vi "whoilbert -- test -- V1.vi"() -> ()   [LabVIEW 2020]
uses:
  publisher action.ctl
panel:
  in  "sweeper panel 4":enum32{"orig"}(tab)
  out "Plot: wsweep window vs ω  2":cluster{dbl[], dbl[]}[](graph)
  in  "sweeper panel 3":enum32{"wform"}(tab)
  out "Plot: wsweep window vs ω":cluster{dbl[], dbl[]}[](graph)
  in  "scale gauge: Plot: wsweep win 2":dbl(slide)=4644576329.775502 min=0.0 max=0.3 step=1e-06 scale=1e-05..50000000000.0 scale format="%#_3p"
  in  "sweeper panel 2":enum32{"main", "parameters"}(tab)
  out "Plot: wsweep window":cluster{dbl[], dbl[]}[](graph)
  in  "scale gauge: Plot: wsweep win":dbl(slide)=4644576329.775502 min=0.0 max=0.3 step=1e-06 scale=1e-05..1000.0 scale format="%#_3p"
  in  "woffset":dbl(slide)=0.6996996996996996 scale=-10.0..10.0
  in  "wrange":dbl=10000.0 format="%#_13g"
  in  "wpoints":i64=100
  in  "ω1":cdb=0.0-40.0i format="%#_13g"
  in  "ω2":cdb=0.0-1.0i format="%#_13g"
  in  "A1":cdb=2.0+0.0i format="%#_13g"
  in  "A2":cdb=1.0+0.0i format="%#_13g"
  in  "κ0":dbl(slide)=5.830000000000001e-10 min=0.0 max=0.3 step=1e-12 scale=1e-10..1e-07 scale format="%#_3p"
  in  "ζ":dbl(slide)=0.003542 min=0.0 max=0.3 step=1e-06 scale=1e-05..10.0 scale format="%#_3p"
  in  "τN":dbl(slide)=0.004864484047644512 min=0.0 max=0.3 step=1e-06 scale=1e-06..10.0 scale format="%#_3p"
  in  "T1":dbl(slide)=0.03855743450772209 min=0.0 max=0.3 step=1e-06 scale=0.0001..10.0 scale format="%#_3p"
  in  "τC":dbl(slide)=0.09541 min=0.0 max=0.3 step=1e-06 scale=1e-05..10.0 scale format="%#_3p"
  in  "τS":dbl(slide)=0.02006412528739728 min=0.0 max=0.3 step=1e-06 scale=0.001..10.0 scale format="%#_3p"
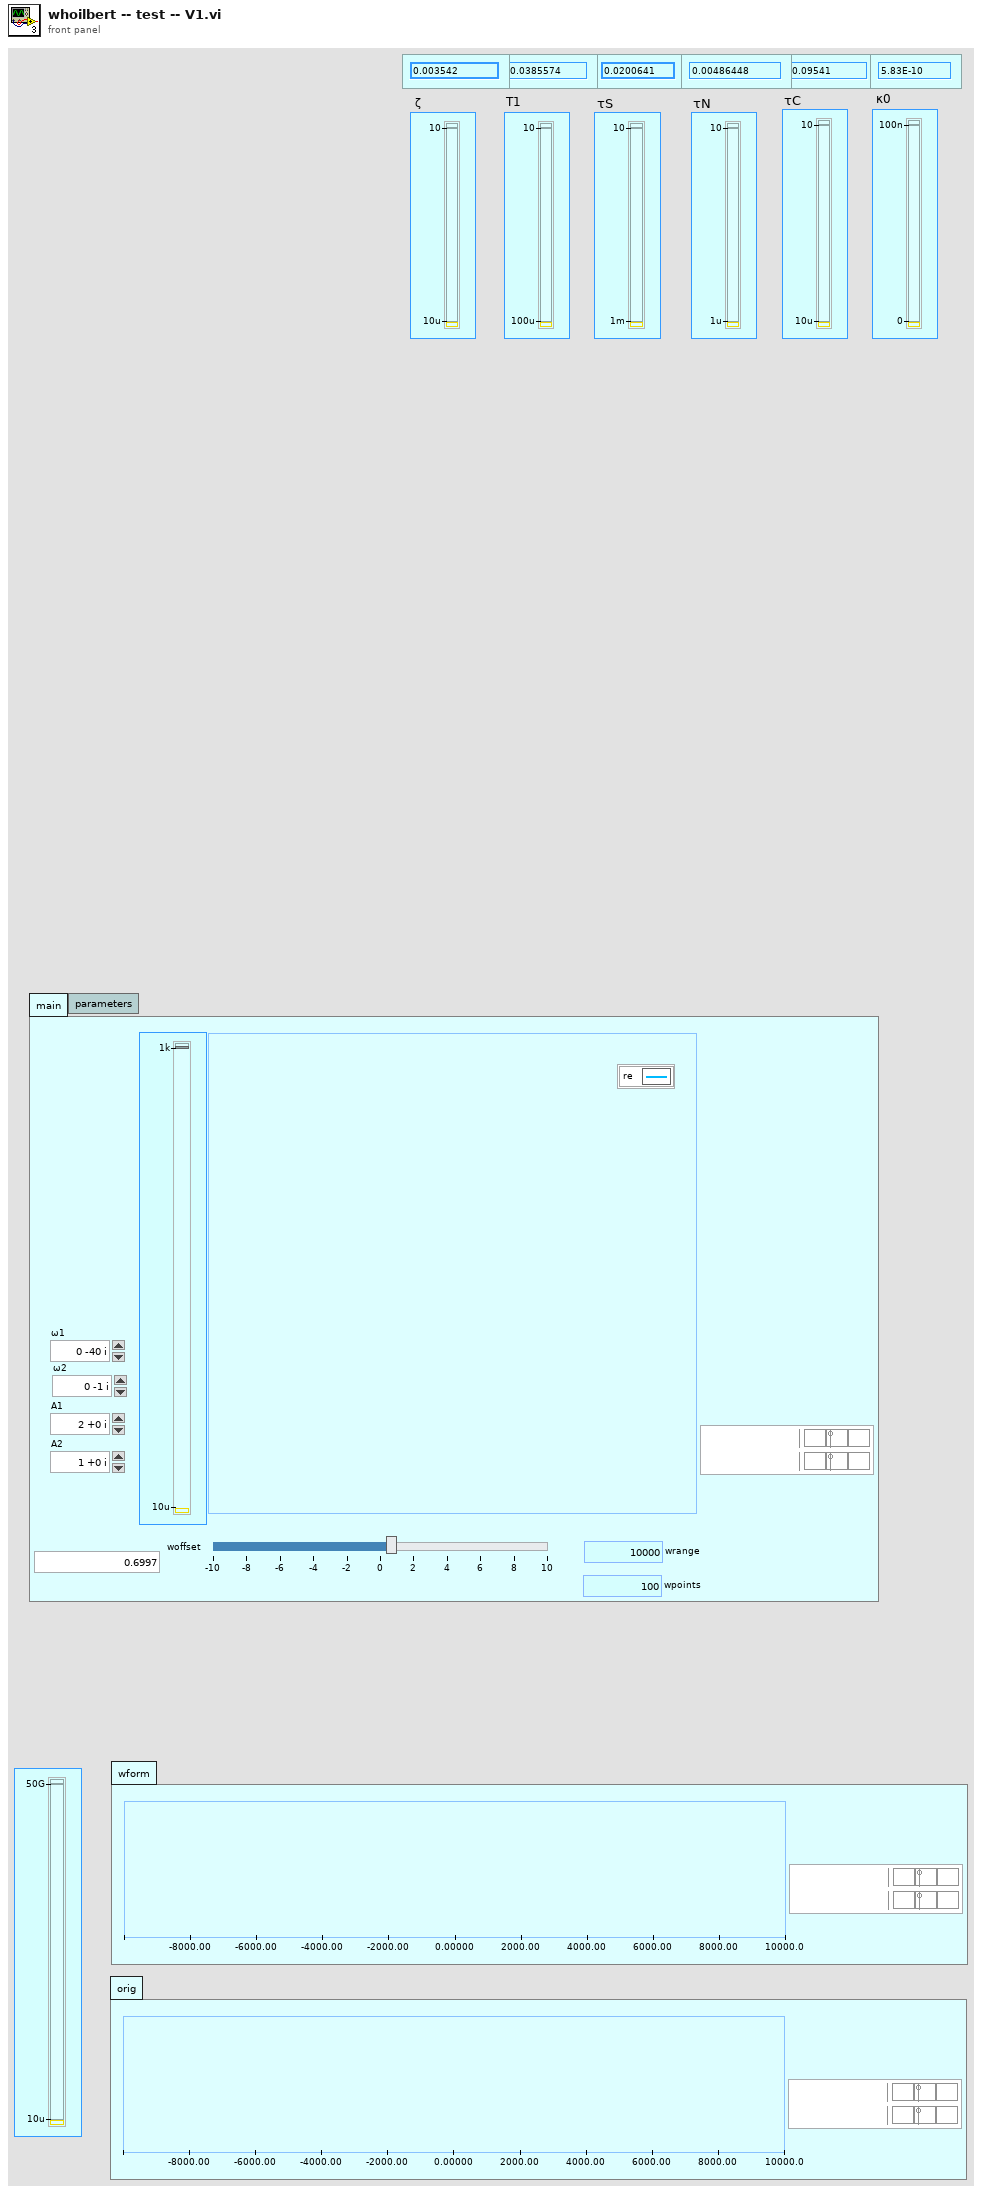
[diagram p1: front panel]
types:
  T1 = typedef "publisher action.ctl" = enum16{"set", "get", "init", "check"}
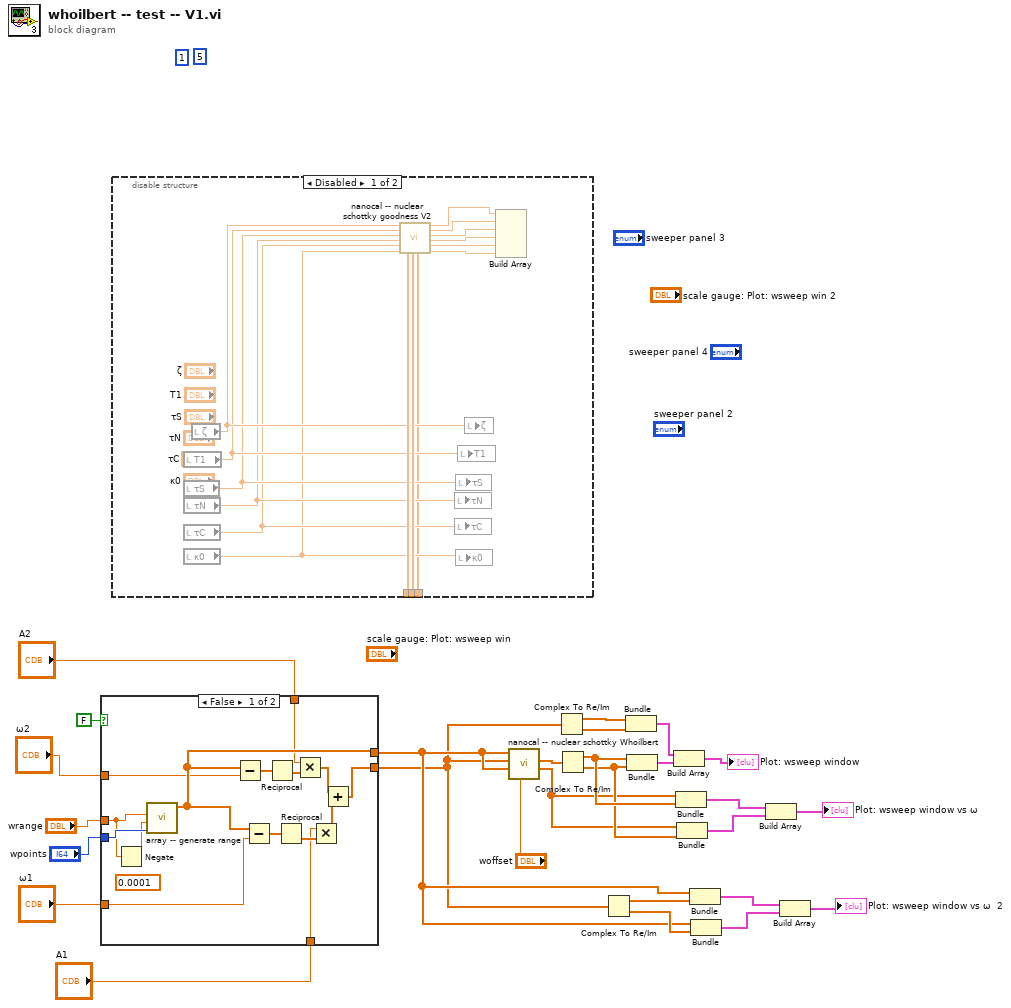
[diagram p0: block diagram]
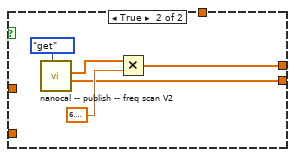
[diagram p2: hidden frame]
diagram:
  (unwired) 5 ("index")
  (unwired) 1
  n1 = case shown="False" FALSE {
    tunnel: [w36 w44] -> w10
    tunnel: [w35 w43] -> w7
    tunnel: "wrange" -> [w33 _]
    tunnel: "wpoints" -> [w34 _]
    tunnel: "ω2" -> [w31 _]
    tunnel: "ω1" -> [w30 _]
    tunnel: "A1" -> [w29 _]
    tunnel: "A2" -> [w28 _]
    frame False {
      (unwired) 0.0001 ("ω from")
      n2 = Negate(x=w33) -> (-x=w32:dbl)
      n3 = call "array -- generate range.vi"("ω points"=w34, "ω from"=w32, "ω to"=w33) -> ("ω out"=w36:dbl[])  [unwired: 8 in]
      n4 = Subtract(x=w36, y=w31) -> (x-y=w41:cdb[])
      n5 = Subtract(x=w36, y=w30) -> (x-y=w42:cdb[])
      n6 = Reciprocal(x=w41) -> (1/x=w40:cdb[])
      n7 = Reciprocal(x=w42) -> (1/x=w39:cdb[])
      n8 = Multiply(x=w28, y=w40) -> (x*y=w37:cdb[])
      n9 = Multiply(x=w29, y=w39) -> (x*y=w38:cdb[])
      n10 = Add(x=w37, y=w38) -> (x+y=w35:cdb[])
    }
    frame True {
      n11 = call "nanocal -- publish -- freq scan V2.vi"("publisher action"=publisher_action."get") -> ("z out (V)"=w43:cdb[], "ω out (Hz)"=w46:dbl[])  [unwired: 8 in, 1 out]
      n12 = Multiply(x=w46, y=6.283185307179586) -> (x*y=w44:dbl[])
    }
  }
  n13 = disable-structure shown="Disabled" {
    disable-tunnel: _ -> [w62 _]
    disable-tunnel: _ -> [w61 _]
    disable-tunnel: _ -> [w54 _]
    frame Disabled {
      n14 = local read "T1"() -> (w59:dbl)
      n15 = local read "τS"() -> (w58:dbl)
      n16 = local read "τN"() -> (w57:dbl)
      n17 = local read "τC"() -> (w56:dbl)
      n18 = local read "κ0"() -> (w55:dbl)
      n19 = local read "ζ"() -> (w60:dbl)
      n20 = call "nanocal -- nuclear schottky goodness V2.vi"("ζ"=w60, "T1"=w59, "τS"=w58, "τN"=w57, "τC"=w56, "κ0"=w55, "ω (rad/sec)"=w62, "Voltage IN (V)"=w61, "dz/dω IN (V)"=w54) -> ("d ln G / d ln ζ"=w53:dbl, "d ln G / d ln τ1"=w52:dbl, "d ln G / d ln τS"=w51:dbl, "d ln G / d ln τN"=w50:dbl, "d ln G / d ln τC"=w49:dbl, "d ln G / d ln κ0"=w48:dbl)  [unwired: 4 in, 1 out]
      n21 = local write "τN"(w57) -> ()
      n22 = local write "τC"(w56) -> ()
      n23 = local write "τS"(w58) -> ()
      n24 = local write "κ0"(w55) -> ()
      n25 = local write "T1"(w59) -> ()
      n26 = local write "ζ"(w60) -> ()
      n27 = Build Array(w53, w52, w51, w50, w49, w48) -> ()  [unwired: 1 out]
    }
    frame Enabled {
    }
  }
  n28 = call "nanocal -- nuclear schottky Whoilbert.vi"("ω shift"="woffset", "new ω IN (rad/sec)"=w10, "Voltage IN (V)"=w7, "ω IN (rad/sec)"=w10) -> ("new ω out (rad/sec)"=w9:dbl[], "Voltage OUT (V)"=w27:cdb[])  [unwired: 5 in, 1 out]
  n29 = Complex To Re/Im(x + iy=w7) -> (x=w8:dbl[], y=w6:dbl[])
  n30 = Complex To Re/Im(x + iy=w27) -> (x=w21:dbl[], y=w20:dbl[])
  n31 = Complex To Re/Im(x + iy=w7) -> (x=w16:dbl[], y=w15:dbl[])
  n32 = Bundle(w8, w6) -> (w5:cluster{dbl[], dbl[]})  [unwired: 1 in]
  n33 = Bundle(w21, w20) -> (w25:cluster{dbl[], dbl[]})  [unwired: 1 in]
  n34 = Build Array(w5, w25) -> (→"Plot: wsweep window":cluster{dbl[], dbl[]}[])
  n35 = Bundle("new ω out (rad/sec)"=w9, w21) -> (w23:cluster{"new ω out (rad/sec)":dbl[], dbl[]})  [unwired: 1 in]
  n36 = Bundle("new ω out (rad/sec)"=w9, w20) -> (w22:cluster{"new ω out (rad/sec)":dbl[], dbl[]})  [unwired: 1 in]
  n37 = Bundle("ω out"=w10, w16) -> (w18:cluster{"ω out":dbl[], dbl[]})  [unwired: 1 in]
  n38 = Bundle("ω out"=w10, w15) -> (w17:cluster{"ω out":dbl[], dbl[]})  [unwired: 1 in]
  n39 = Build Array(w23, w22) -> (→"Plot: wsweep window vs ω":cluster{"new ω out (rad/sec)":dbl[], dbl[]}[])
  n40 = Build Array(w18, w17) -> (→"Plot: wsweep window vs ω  2":cluster{"ω out":dbl[], dbl[]}[])
